vi "zmq_ctx_destroy.vi"(3 "error in":errorcluster, 4 "reap? (F)":bool, 5 "context in":refnum<class "zmq_context.lvclass">) -> (0 "error out":errorcluster)   [LabVIEW 2019, in "zeromq.lvlib" / "zmq_context.lvclass"]
doc: "Terminates the <b>context</b> fed in. This is a <b>blocking</b> call, and only returns once every socket associated with the context has been terminated.\n\nBecause operations may be pending on sockets, they are given some time (ZMQ_LINGER) to finish before being shut-down by the term call.\n\nThis behaviour can be overwritten by setting <b>reap?</b> to True, which will eliminate all sockets opened by LabVIEW in this context immediately without worrying about close/blocking operations. This may result in unexpected data loss and should only be used in abort situations.\n\nDetailed API documentation: http://api.zeromq.org/3-2:zmq-ctx-destroy"
uses:
  zmq_context.lvclass
  zmq_context.lvclass/zmq_context.ctl
  <vilib>/Utility/error.llb/Error Cluster From Error Code.vi
  zeromq.lvlib
panel:
  # "ØMQ"
  # "labview"
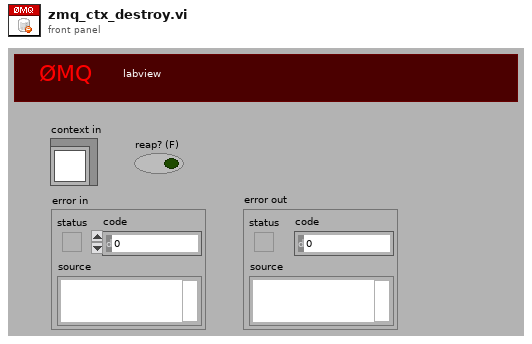
[diagram p1: front panel]
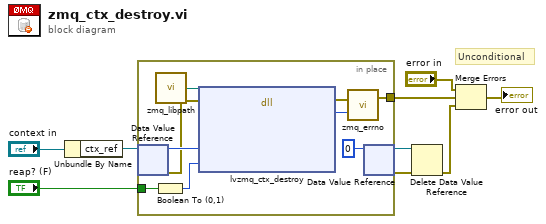
[diagram p0: block diagram]
diagram:
  # "Unconditional"
  n1 = Unbundle By Name("context in") -> ("ctx_ref"=w7:refnum<data-value>)
  n2 = in-place {
    in-place-border: [w16] -> w9
    in-place-border: "reap? (F)" -> [w14]
    n3 = in-place-dvr #1(w7) -> (w15:u64, w10:errorcluster)
    n4 = Boolean To (0,1)(Boolean=w14) -> (0, 1=w13:i16)
    n5 = call "zmq_libpath.vi"() -> ("path"=w11:path)
    n6 = dll-call lib="?" fn="lvzmq_ctx_destroy" ("zmq_labview.dll:lvzmq_term")(path in=w11, error in=w10, "ctx_obj"=w15, "flags"=w13) -> (error out=w17:errorcluster, "return"=w18:i32)  [unwired: 5 in, 1 out]
    n7 = call "zmq_errno.vi"("retval"=w18, "error in"=w17) -> ("error out"=w16:errorcluster)  [unwired: 1 out]
    n8 = in-place-dvr #1(u64 0 ("data value")) -> (w4:refnum<data-value>, w5:errorcluster)
  }
  n9 = Delete Data Value Reference(data value reference=w4, error in=w5) -> (error out=w1:errorcluster)  [unwired: 1 out]
  n10 = Merge Errors("error in", w9, w1) -> (→"error out":errorcluster)
